vi "Read Text.vi"(9 "Path in":refnum<class "Path.lvclass">) -> (3 "Path out":refnum<class "Path.lvclass">, 4 "Text":refnum<class "Text.lvclass">)   [LabVIEW 2014, in "Raspberry Pi Compatible Compiler for LabVIEW.lvlib" / "Path.lvclass"]
uses:
  Path.lvclass
  Text/Text.lvclass
  Path.lvclass/Path.ctl
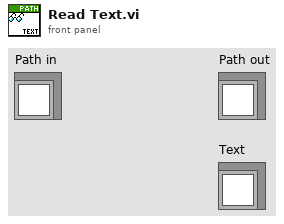
[diagram p1: front panel]
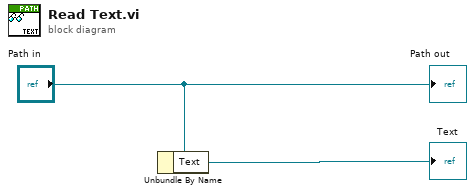
[diagram p0: block diagram]
diagram:
  n1 = Unbundle By Name("Path in") -> ("Text"=→"Text":refnum<class "Text.lvclass">)
  "Path out" <- "Path in"
